vi "testUDP.vi"() -> ()   [LabVIEW 2016]
uses:
  <vilib>/userdefined/High Color/IMAQdx.ctl
  <vilib>/vision/driver/NI_Vision_Acquisition_Software.lvlib
panel:
  out "appended array":u32[](array[numeric])
  out "millisecond timer value":u32
  in  "Camera":T1="cam0"
  # "Overview: Demonstrates how to acquire an image from a camera using the IMAQdx API, transfer the image to a FPGA target for processing, and retrieve the processed image for display or further processing on the host.\nRequirements:\n- LabVIEW FPGA\n- Vision Acquisition Software\n- Vision Development Module\nInstructions:\n1. Select a Camera\n2. Run the VI."
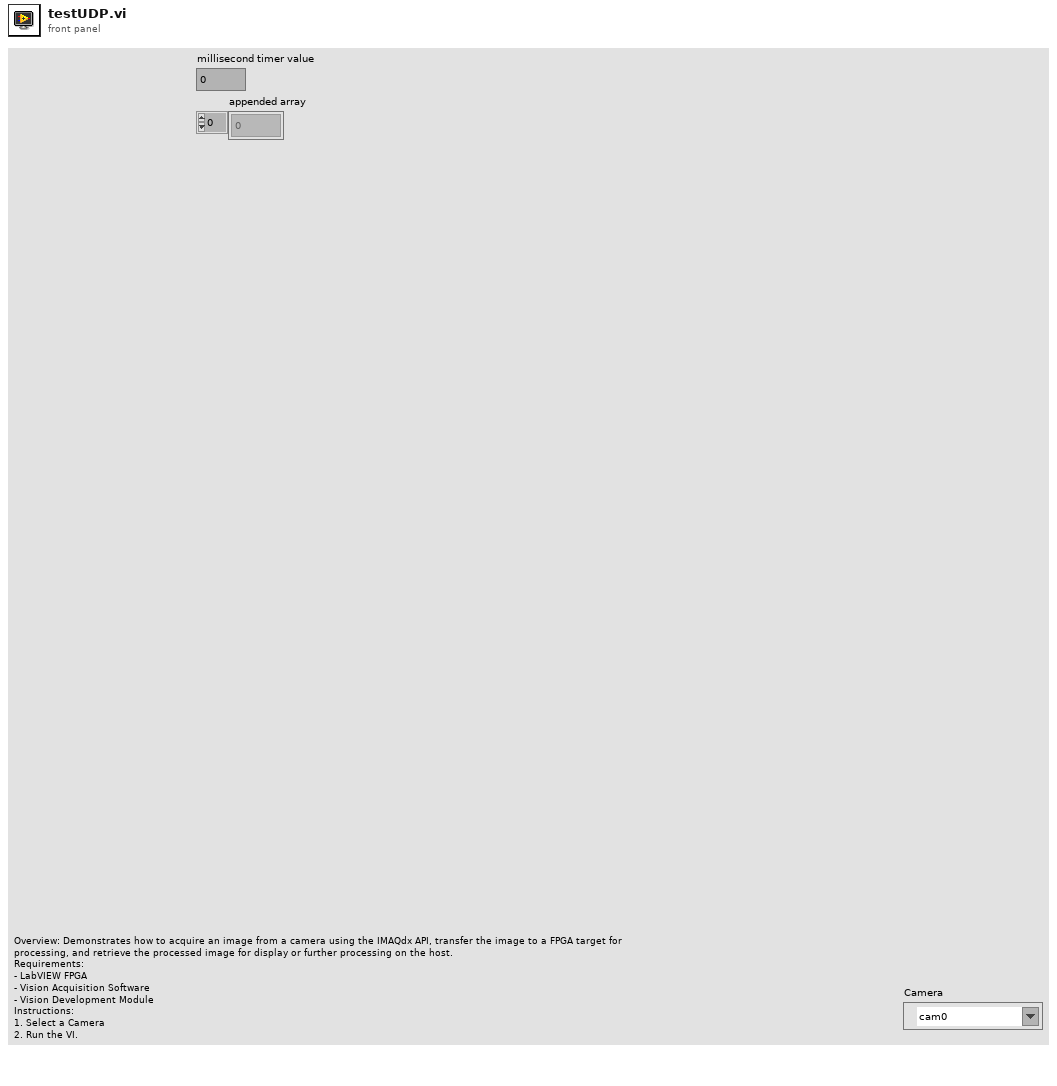
[diagram p1: front panel]
types:
  T1 = typedef "IMAQdx.ctl" = refnum<k21>
  T2 = typedef "Image Type" = u32
  T3 = typedef "IMAQ Image.ctl" = refnum<image>
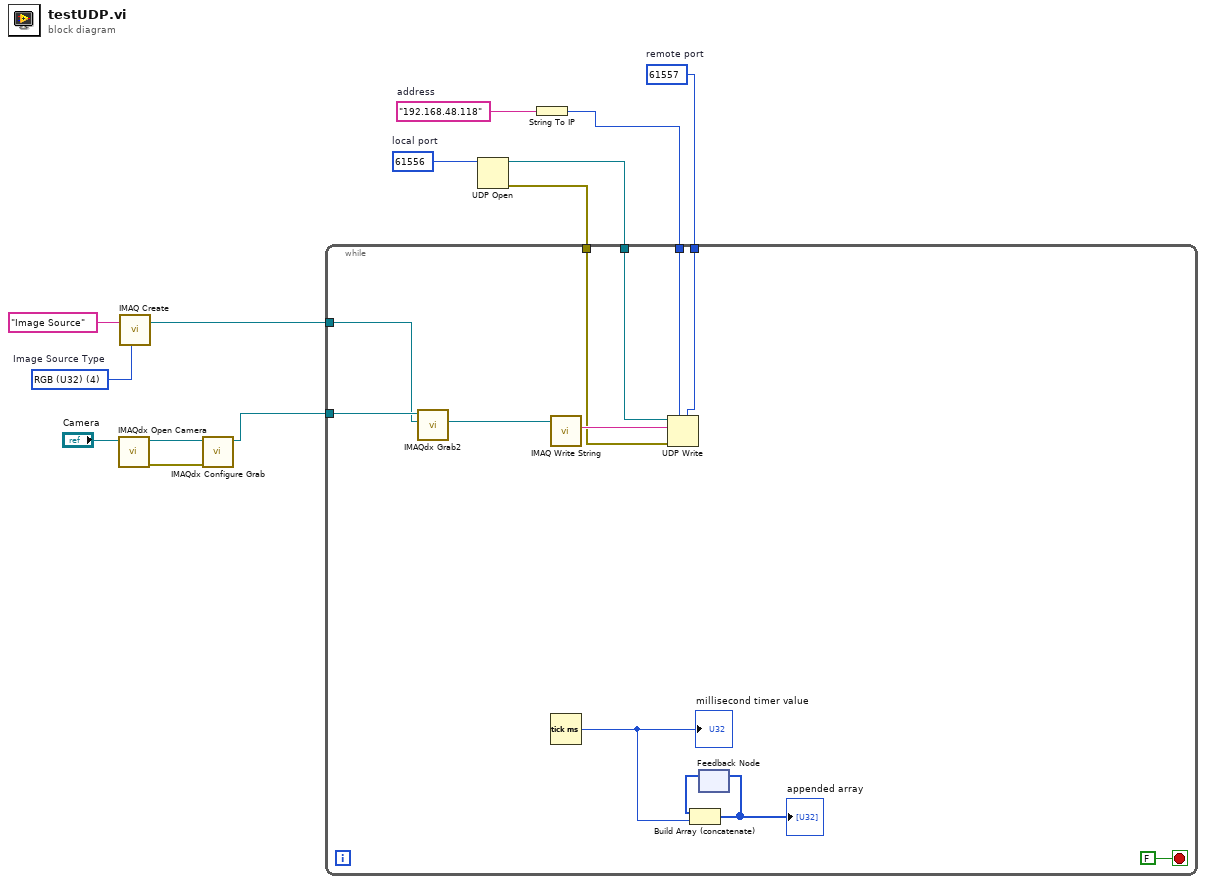
[diagram p0: block diagram]
diagram:
  w3 = "192.168.48.118"  # address
  w6 = u16 61556  # local port
  w1 = u16 61557  # remote port
  w12 = T2 4 items=["Grayscale (U8)", "Grayscale (I16)", "Grayscale (SGL)", "Complex (CSG)", "RGB (U32)", "HSL (U32)", "RGB (U64)", "Grayscale (U16)"]  # Image Source Type
  n1 = call <vilib>:"IMAQdx Open Camera.vi"("Session In"="Camera") -> ("error out"=w9:errorcluster, "Session Out"=w10:T1)  [unwired: 9 in]
  n2 = call "IMAQ Create"("Image Name"="Image Source", "Image Type"=w12) -> ("New Image"=w7:T3)  [unwired: 3 in, 1 out]
  n3 = call <vilib>:"IMAQdx Configure Grab.vi"("error in"=w9, "Session In"=w10) -> ("Session Out"=w8:T1)  [unwired: 8 in, 1 out]
  n4 = UDP Open(11:w6) -> (port=w5:refnum<k16>, 0:w4:errorcluster)  [unwired: 4 in, 1 out]
  n5 = String To IP(1:w3) -> (0:w2:u32)
  n6 = while {
    tunnel: w8 -> [w25]
    tunnel: w7 -> [w24]
    tunnel: w5 -> [w21]
    tunnel: w4 -> [w20]
    tunnel: w2 -> [w19]
    tunnel: w1 -> [w18]
    stop <- FALSE stop-if-true
    n7 = call <vilib>:"IMAQdx Grab2.vi"("Image In"=w24, "Session In"=w25) -> ("Image Out"=w22:T3)  [unwired: 6 in, 3 out]
    n8 = call-poly "IMAQ Write String"("Image"=w22) -> ("FileString"=w23:string)  [unwired: 8 in, 2 out]
    n9 = Tick Count (ms)() -> (millisecond timer value=w16:u32)
    "millisecond timer value" <- w16
    n10 = UDP Write(address=w19, port or service name=w18, connection ID=w21, data in=w23, 8:w20) -> ()  [unwired: 1 in, 2 out]
    n11 = feedback #1() -> (w14:u32[])  [unwired: 1 in]
    n12 = Build Array (concatenate)(w14, w16) -> (w15:u32[])
    "appended array" <- w15
    n13 = feedback-in #1(w15) -> ()
  }
